vi "dante.vi"() -> ()   [LabVIEW 2019]
panel:
  in  "Tank":dbl(slide) scale=0.0..10.0
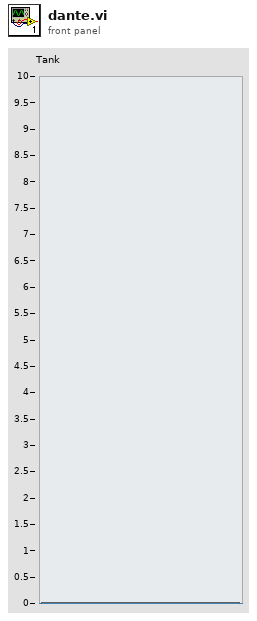
[diagram p1: front panel]
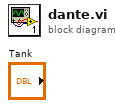
[diagram p0: block diagram]
diagram:
